vi "Untitled 3.vi"() -> ()   [LabVIEW 2020]
uses:
  Global 3.vi
panel:
  in  "stop":bool
  in  "Boolean 2":bool
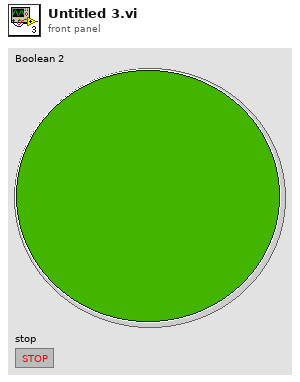
[diagram p1: front panel]
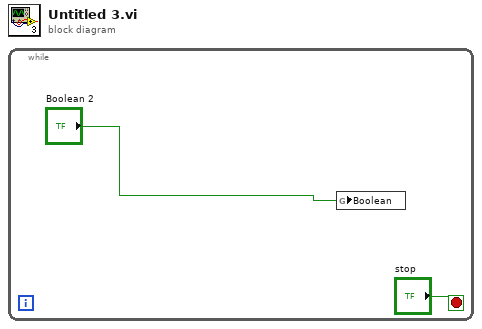
[diagram p0: block diagram]
diagram:
  n1 = while {
    stop <- "stop" stop-if-true
    n2 = global write "Global 3.vi" "Boolean"("Boolean 2") -> ()
  }
